vi "Property_Always Refresh.vi"(8 "error in (no error)":errorcluster, 11 "Dependency Source_Custom in":refnum<class "Dependency Source_Custom.lvclass">) -> (0 "error out":errorcluster, 2 "Always Refresh Targets?":bool, 3 "Dependency Source_Custom out":refnum<class "Dependency Source_Custom.lvclass">)   [LabVIEW 2019, in "Project.Dependencies Finder.lvlib" / "Dependency Source_Custom.lvclass"]
doc: "Set this property to override the refresh behaviour. If True the Dependency Source will be skipped on 'Refresh Target' but always refreshed when finding dependencies.\n\nThis implementation returns True."
uses:
  Dependency Source_Custom.lvclass
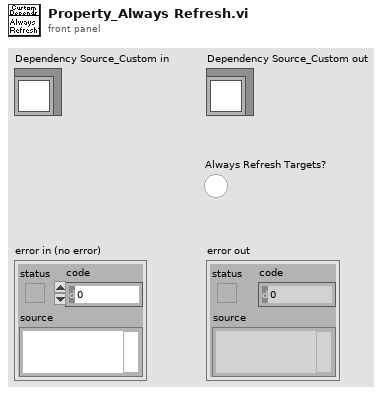
[diagram p1: front panel]
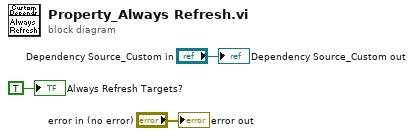
[diagram p0: block diagram]
diagram:
  "error out" <- "error in (no error)"
  "Dependency Source_Custom out" <- "Dependency Source_Custom in"
  "Always Refresh Targets?" <- TRUE ("Always Refresh Targets?")
